vi "Read Element.vi"(8 "error in (no error)":errorcluster, 11 "Array Element 1D in":refnum<class "Vector of Elements.lvclass">) -> (0 "error out":errorcluster, 2 "Element.lvclass":refnum<class "Abs_Type.lvclass">, 3 "Array Element 1D out":refnum<class "Vector of Elements.lvclass">)   [LabVIEW 2021, in "Vector of Elements.lvclass"]
uses:
  Vector of Elements.lvclass
  C:/Users/Tim/Documents/LabVIEW/2021/Data Classes/Source/Element/Vector Parent/Vector Parent.lvclass
  Abs_Types/Type/Abs_Type.lvclass
  Element/Vector Parent/Vector Parent.lvclass/Vector Parent.ctl
  Vector of Elements.lvclass/Vector of Elements.ctl
  Element/Vector Parent/Properties/Read Index.vi
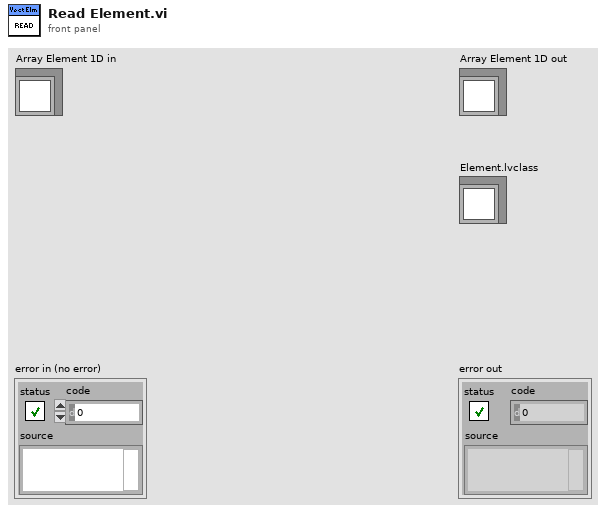
[diagram p1: front panel]
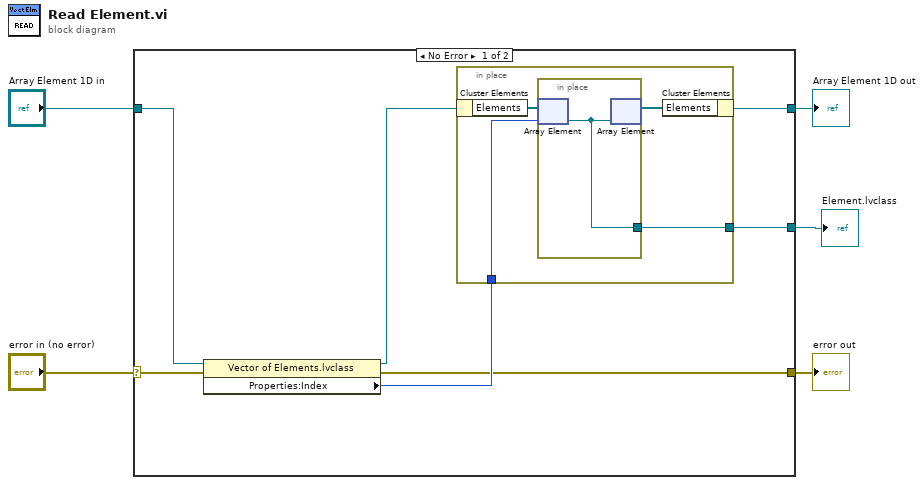
[diagram p0: block diagram]
diagram:
  n1 = case shown="No Error" "error in (no error)" {
    selector: "error in (no error)" -> [w11 w19]
    tunnel: [w9 w19] -> w4
    tunnel: [w6 w18] -> w2
    tunnel: "Array Element 1D in" -> [w12 w18]
    tunnel: [w8 _] -> w1
    frame No Error {
      n2 = property class="Vector of Elements.lvclass"(reference=w12, error in=w11) -> (reference out=w7:refnum<class "Vector of Elements.lvclass">, error out=w9:errorcluster, "Properties:Index"=w10:i32)
      n3 = in-place {
        in-place-border: w10 -> [w15]
        in-place-border: [w14] -> w8
        n4 = in-place-cluster #1(w7) -> ("Elements"=w16:refnum<class "Abs_Type.lvclass">[])
        n5 = in-place {
          in-place-border: [w17] -> w14
          n6 = in-place-array #2(w16, w15) -> (w17:refnum<class "Abs_Type.lvclass">)
          n7 = in-place-array #2(w17) -> (w13:refnum<class "Abs_Type.lvclass">[])  [unwired: 1 out]
        }
        n8 = in-place-cluster #1("Elements"=w13) -> (w6:refnum<class "Vector of Elements.lvclass">)
      }
    }
    frame Error {
    }
  }
  "error out" <- w4
  "Array Element 1D out" <- w2
  "Element.lvclass" <- w1
